vi "create tag select channels.vi"(9 "data type":T1, 10 "tag select name":string) -> (0 "created channels":refnum<class "TBM channel.lvclass">[](array[class]), 1 "inputs":refnum<class "TBM channel.lvclass">[](array[class]), 2 "select":refnum<class "TBM channel.lvclass">, 3 "output":refnum<class "TBM channel.lvclass">)   [LabVIEW 2013, in "current tag file io module configuration.lvclass"]
uses:
  current tag file io module configuration.lvclass
  <vilib>/NI/Tag Bus Module Framework/channel/TBM channel.lvclass
  <vilib>/NI/Tag Bus/tag/Data Type.ctl
  <vilib>/NI/Tag Bus Module Framework/channel/channel classification.ctl
  <vilib>/NI/Tag Bus/tag/tag descriptor.lvclass
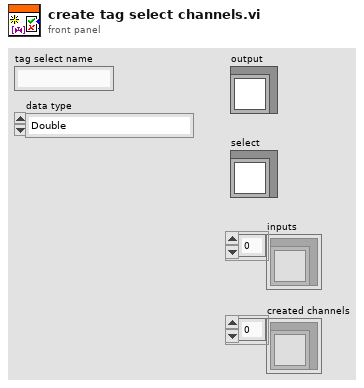
[diagram p1: front panel]
types:
  T1 = typedef "tag bus.lvlib/tag descriptor.lvclass/Data Type.ctl" = enum16{"Double", "Single", "I64", "I32", "I16", "I8", "U64", "U32", "U16", "U8", "Boolean", "String", "Array of Double", "Array of Single", "Array of I64", "Array of I32", "Array of I16", "Array of I8", "Array of U64", "Array of U32", "Array of U16", "Array of U8", "Array of Boolean", "Array of String"}
  T2 = typedef "TBM channel.lvclass/channel classification.ctl" = enum16{"input data", "output data", "processing parameter", "processing result"}
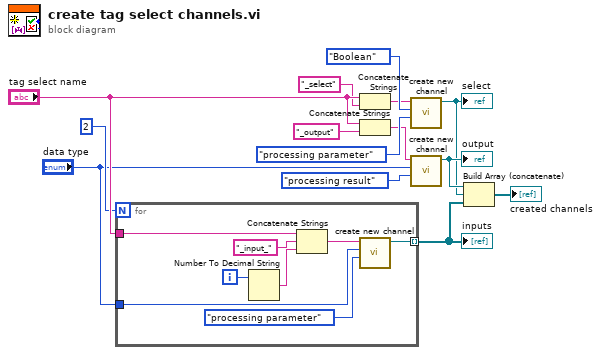
[diagram p0: block diagram]
diagram:
  n1 = for {
    N: 2 -> [_]
    tunnel: "tag select name" -> [w19]
    tunnel: [w16] -> w14 mode=indexing
    tunnel: "data type" -> [w15]
    i -> [w18]
    n2 = Number To Decimal String(number=w18) -> (decimal integer string=w17:string)  [unwired: 1 in]
    n3 = Concatenate Strings(w19, "_input_" ("string"), w17) -> (w21:string)
    n4 = call <vilib>:"create new channel.vi"("channel classification"=channel_classification."processing parameter", "data type"=w15, "channel name"=w21) -> ("channel"=w16:refnum<class "TBM channel.lvclass">)  [unwired: 8 in]
  }
  "inputs" <- w14
  n5 = Concatenate Strings("tag select name", "_select" ("string")) -> (w4:string)
  n6 = Concatenate Strings("tag select name", "_output" ("string")) -> (w7:string)
  n7 = call <vilib>:"create new channel.vi"("channel classification"=channel_classification."processing parameter", "data type"=Data_Type."Boolean", "channel name"=w4) -> ("channel"=w1:refnum<class "TBM channel.lvclass">)  [unwired: 8 in]
  "select" <- w1
  n8 = call <vilib>:"create new channel.vi"("channel classification"=channel_classification."processing result", "data type"="data type", "channel name"=w7) -> ("channel"=w2:refnum<class "TBM channel.lvclass">)  [unwired: 8 in]
  "output" <- w2
  n9 = Build Array (concatenate)(w2, w1, w14) -> (→"created channels":refnum<class "TBM channel.lvclass">[])
